vi "solar_log EnQ (Message).vi"(4 "Clear Error? (T)":bool=TRUE, 6 "Type (CMD)":enum8{"CMD", "TLM"}(ring), 7 "LogIgnore":string[](array[string]), 8 "error in (no error)":errorcluster, 9 "DATA":variant, 10 "MSG":string, 11 "Target":string) -> (0 "error out":errorcluster)   [LabVIEW 2018]
doc: "This enqueues a log message to the logger process in human readable format: 'TARGET:PACKET{VALUE,VALUE,...}'. <b>Log Ignore</b> filters messages to log using wildcards ('*')."
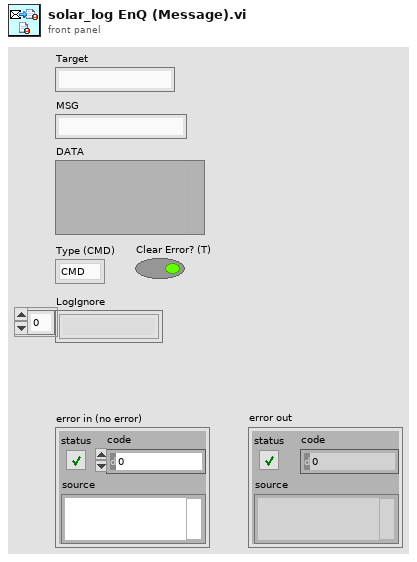
[diagram p1: front panel]
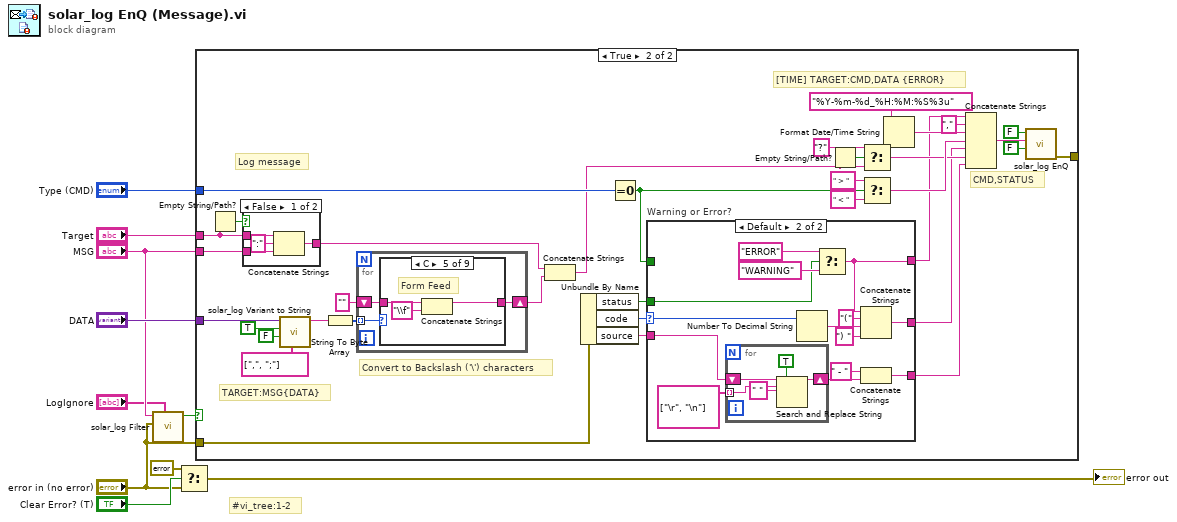
[diagram p0: block diagram]
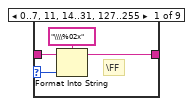
[diagram p3: hidden frame]
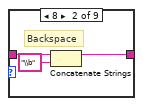
[diagram p4: hidden frame]
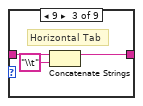
[diagram p5: hidden frame]
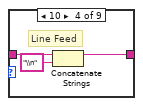
[diagram p6: hidden frame]
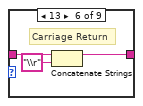
[diagram p7: hidden frame]
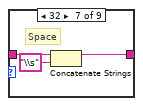
[diagram p8: hidden frame]
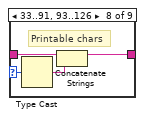
[diagram p9: hidden frame]
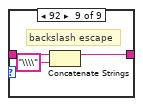
[diagram p10: hidden frame]
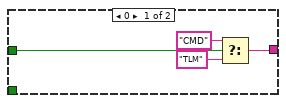
[diagram p12: hidden frame]
diagram:
  # "#vi_tree:1-2"
  n1 = call "solar_log Filter.vi"("LogIgnore"="LogIgnore", "error in (no error)"="error in (no error)", "MSG"="MSG") -> ("Log?"=w2:bool)  [unwired: 8 in]
  n2 = Select(t=errorcluster {"status"=FALSE, "code"=0, "source"=""}, s="Clear Error? (T)", f="error in (no error)") -> (s? t:f=→"error out":errorcluster)
  n3 = case shown="True" w2 {
    tunnel: "DATA" -> [_ w24]
    tunnel: "MSG" -> [_ w43]
    tunnel: "Target" -> [_ w44]
    tunnel: "Type (CMD)" -> [_ w41]
    tunnel: "error in (no error)" -> [_ w17]
    tunnel: [_ w16] -> _
    frame False {
    }
    frame True {
      # "Convert to Backslash ('\\') characters"
      # "Log message"
      # "CMD,STATUS"
      # "[TIME] TARGET:CMD,DATA {ERROR}"
      # "TARGET:MSG{DATA}"
      n4 = Empty String/Path?(string/path=w44) -> (empty?=w45:bool)
      n5 = case shown="False" w45 {
        tunnel: w44 -> [w81 _]
        tunnel: w43 -> [w80 w82]
        tunnel: [w78 w82] -> w42
        frame False {
          n6 = Concatenate Strings(w81, ":" ("string"), w80) -> (w78:string)
        }
        frame True {
        }
      }
      n7 = call "solar_log Variant to String.vi"("ArrayDelimiters (1D,2D)"=string[] [",", ";"], "Boolean as 0,1? (F)"=FALSE, "Use Enum Names? (F)"=TRUE, "Variant"=w24) -> ("String"=w12:string)  [unwired: 5 in, 2 out]
      n8 = String To Byte Array(string=w12) -> (unsigned byte array=w14:u8[])
      n9 = for {
        tunnel: w14 -> [w48] mode=indexing
        shift-right: [w47] -> w11
        shift-left: "" -> [w46]
        n10 = case shown="C" w48 {
          selector: w48 -> [w52 _ _ _ _ _ _ w72 _]
          tunnel: [w50 w54 w57 w60 w63 w66 w69 w73 w76] -> w47
          tunnel: w46 -> [w49 w55 w58 w61 w64 w67 w70 w74 w77]
          frame 0..7, 11, 14..31, 127..255 {
            # "\\FF"
            n11 = Format Into String(format string="\\\\%02x", initial string=w49, w52) -> (resulting string=w50:string)  [unwired: 1 in, 1 out]
          }
          frame 8 {
            # "Backspace"
            n12 = Concatenate Strings(w55, "\\b" ("string")) -> (w54:string)
          }
          frame 9 {
            # "Horizontal Tab"
            n13 = Concatenate Strings(w58, "\\t" ("string")) -> (w57:string)
          }
          frame 10 {
            # "Line Feed"
            n14 = Concatenate Strings(w61, "\\n" ("string")) -> (w60:string)
          }
          frame 12 {
            # "Form Feed"
            n15 = Concatenate Strings(w64, "\\f" ("string")) -> (w63:string)
          }
          frame 13 {
            # "Carriage Return"
            n16 = Concatenate Strings(w67, "\\r" ("string")) -> (w66:string)
          }
          frame 32 {
            # "Space"
            n17 = Concatenate Strings(w70, "\\s" ("string")) -> (w69:string)
          }
          frame 33..91, 93..126 {
            # "Printable chars"
            n18 = Type Cast(x=w72) -> (*(type *) &x=w71:string)  [unwired: 1 in]
            n19 = Concatenate Strings(w74, w71) -> (w73:string)
          }
          frame 92 {
            # "backslash escape"
            n20 = Concatenate Strings(w77, "\\\\" ("string")) -> (w76:string)
          }
        }
      }
      n21 = Concatenate Strings(w42, w11) -> (w15:string)
      n22 = Unbundle By Name(w17) -> ("status"=w20:bool, "code"=w19:i32, "source"=w18:string)
      n23 = Equal To 0?(x=w41) -> (x = 0?=w37:bool)
      n24 = case "Warning or Error?" shown="Default" w19 {
        selector: w19 -> [_ w96]
        tunnel: w20 -> [_ w93]
        tunnel: [_ w94] -> w32
        tunnel: [w86 w87] -> w29
        tunnel: w18 -> [_ w90]
        tunnel: [_ w91] -> w33
        tunnel: w37 -> [w85 _]
        frame 0 {
          n25 = Select(t="CMD", s=w85, f="TLM") -> (s? t:f=w86:string)
        }
        frame Default {
          n26 = for {
            shift-right: [w103] -> w89
            shift-left: w90 -> [w104]
            tunnel: string[] ["\r", "\n"] -> [w102] mode=indexing
            n27 = Search and Replace String(replace all?=TRUE ("replace all? (F)"), input string=w104, search string=w102, replace string=" " ("replace string (\"\")")) -> (result string=w103:string)  [unwired: 4 in, 3 out]
          }
          n28 = Number To Decimal String(number=w96) -> (decimal integer string=w95:string)  [unwired: 1 in]
          n29 = Select(t="ERROR", s=w93, f="WARNING") -> (s? t:f=w87:string)
          n30 = Concatenate Strings(w87, "(" ("string"), w95, ") " ("string")) -> (w94:string)
          n31 = Concatenate Strings(" - " ("string"), w89) -> (w91:string)
        }
      }
      n32 = Empty String/Path?(string/path=w15) -> (empty?=w34:bool)
      n33 = Select(t="?", s=w34, f=w15) -> (s? t:f=w36:string)
      n34 = Select(t=" > ", s=w37, f=" < ") -> (s? t:f=w40:string)
      n35 = Format Date/Time String(time format string (%c)="%Y-%m-%d_%H:%M:%S%3u" ("format string")) -> (date/time string=w31:string)  [unwired: 2 in]
      n36 = Concatenate Strings(w29, "," ("string"), w31, w40, w32, w36, w33) -> (w26:string)
      n37 = call "solar_log EnQ.vi"("Front? (F)"=FALSE, "MSG"=w26, "Create? (F)"=FALSE) -> ("error out"=w16:errorcluster)  [unwired: 6 in, 2 out]
    }
  }
